vi "Launcher.vi"   [LabVIEW 2021]
uses:
  <vilib>/MGI/Panel Manager/Panel Actor/Panel Actor/Panel Actor.lvclass
  <vilib>/MGI/Panel Manager/Panel Actor/Panel Actor/Launch Root Panel Window.vi
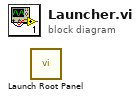
[diagram p0: block diagram]
diagram:
  n1 = call-poly <vilib>:"Launch Root Panel.vi"() -> ()  [unwired: 10 in, 2 out]
